vi "ini_sesion.vi"(8 "error in (no error)":errorcluster, 11 "pulse_gen_and_detect_p2p in":refnum<class "pulse_gen_and_detect_p2p.lvclass">) -> (0 "error out":errorcluster, 3 "pulse_gen_and_detect_p2p out":refnum<class "pulse_gen_and_detect_p2p.lvclass">)   [LabVIEW 2021, in "pulse_gen_and_detect_p2p.lvclass"]
uses:
  pulse_gen_and_detect_p2p.lvclass
  pulse_gen_and_detect_p2p.lvclass/pulse_gen_and_detect_p2p.ctl
  <instrlib>/niRFSG/niRFSG.llb/niRFSG Ref Clock Sources.ctl
  <instrlib>/niRFSA/niRFSA.llb/niRFSA Acquisition Types.ctl
  <vilib>/FPGAPlugInAG/PXIe-5785 (KU060)/niLvFpga_Open_PXIe-5785 (KU060).vi
  <vilib>/rvi/interface/common/dynamic/niFpgaDynamicAddResources.vi
  <vilib>/FPGAPlugInAG/Dynamic/niLvFpga_P2PGetEndpoint_Dynamic.vi
  <vilib>/Utility/error.llb/Error Cluster From Error Code.vi
  <vilib>/rvi/interface/common/niFpgaWaitOnOcc.vi
  <vilib>/rvi/errors/niLvFpgaAdjustHostInterfaceError.vi
  <vilib>/rvi/interface/nirviOpenFPGA/nirviOpenFPGA.xnode
  FPGA Bitfiles/5785_p2p_IQ_gen_1_6GHz_max_and_pulse_detector.lvbitx
  <vilib>/rvi/interface/nirviMethod/nirviMethod.xnode
  <vilib>/rvi/interface/nirviReadWriteControl/nirviReadWriteControl.xnode
  <vilib>/rvi/errors/niLvFpgaMergeErrorWithErrorCode.vi
  <vilib>/rvi/interface/Simulation/niFpgaSimulationCallBeginRW.vi
  <vilib>/FPGAPlugInAG/Dynamic/niLvFpga_StopFifo_Dynamic.vi
  <vilib>/FPGAPlugInAG/Dynamic/niLvFpga_ConfigureFifo_Dynamic.vi
  NiFpgaLv.dll
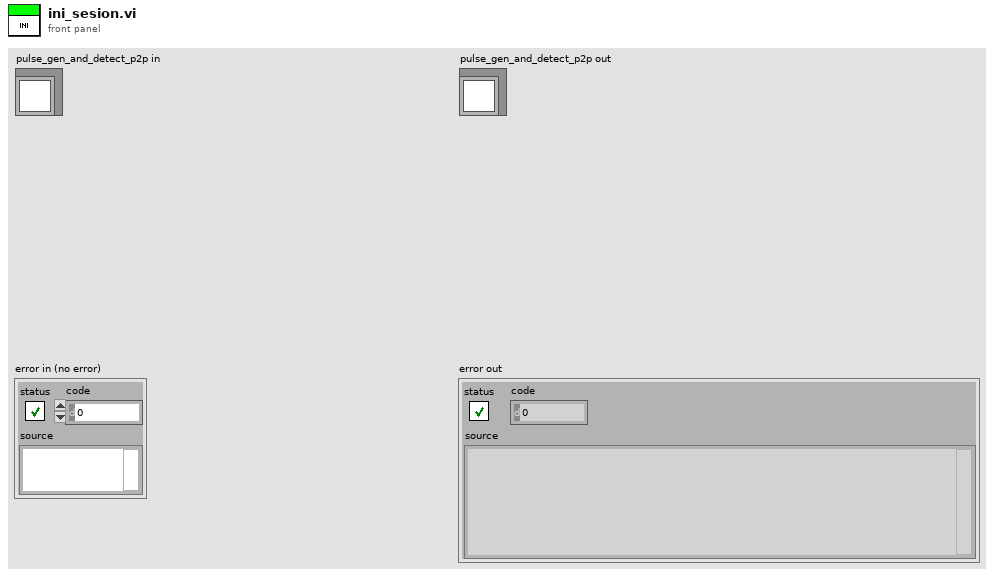
[diagram p1: front panel]
types:
  T1 = typedef "nirio_resource_hc.ctl" = tag
  T2 = cluster{"min PW (fft cycels)":u16, "max PW (fft cycels)":u16, "max gap (fft cycels)":u8, "detection bar (liniar amp)":fxp<+,64,63>, "peak detect":bool}
  T3 = enum16{"open", "open or create", "create or replace", "create", "open (read-only)"}
  T4 = typedef "niRFSG Ref Clock Sources.ctl" = string
  T5 = typedef "niRFSA Acquisition Types.ctl" = i32
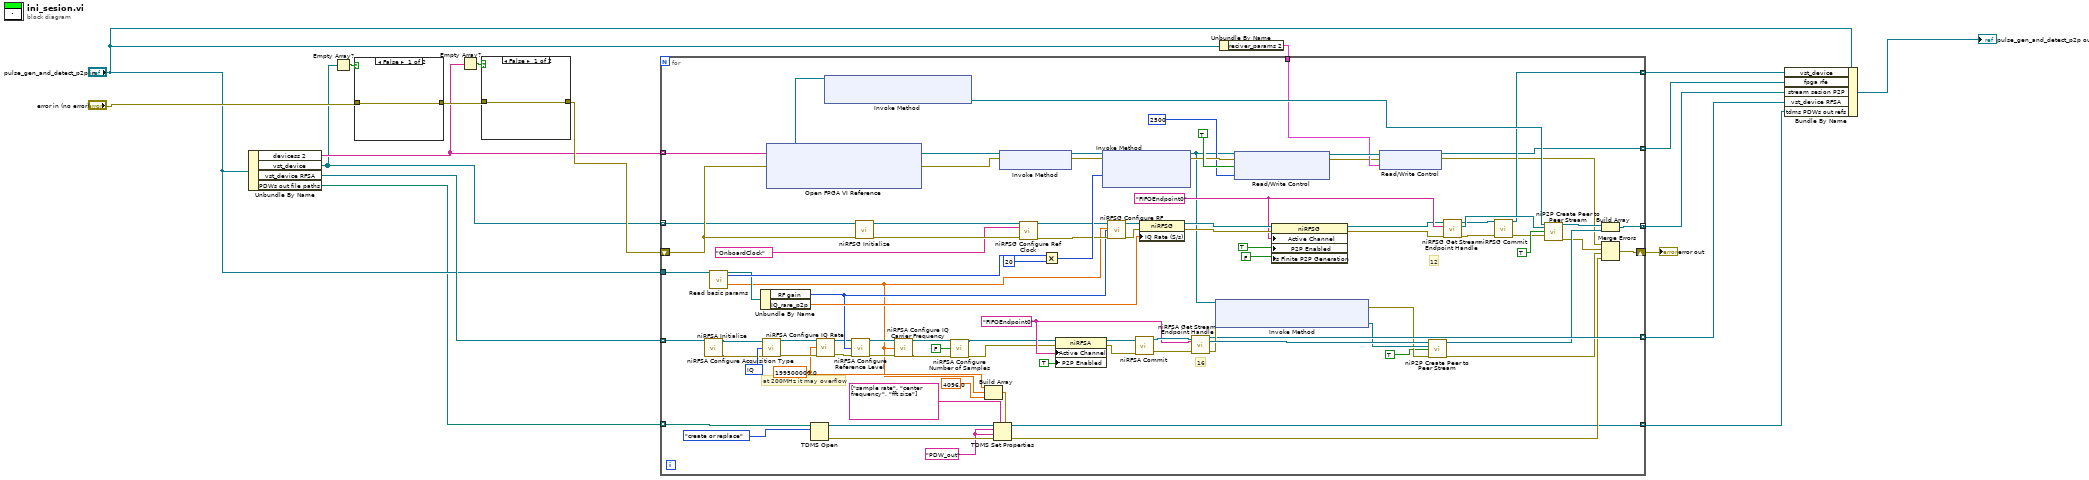
[diagram p0: block diagram]
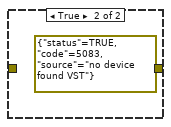
[diagram p2: hidden frame]
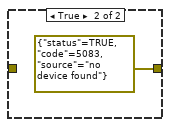
[diagram p3: hidden frame]
diagram:
  n1 = Unbundle By Name("pulse_gen_and_detect_p2p in") -> ("devicess 2"=w12:T1[], "vst_device"=w11:refnum<k15>[], "vst_device RFSA"=w7:refnum<k15>[], "PDWs out file paths"=w3:path[])
  n2 = Empty Array?(array=w11) -> (empty?=w17:bool)
  n3 = case shown="False" w17 {
    tunnel: [w19 errorcluster {"status"=TRUE, "code"=5083, "source"="no device found VST"} ("error in (no error)")] -> w16
    tunnel: "error in (no error)" -> [w19 _]
    frame False {
    }
    frame True {
    }
  }
  n4 = Empty Array?(array=w12) -> (empty?=w18:bool)
  n5 = case shown="False" w18 {
    tunnel: [w21 errorcluster {"status"=TRUE, "code"=5083, "source"="no device found"} ("error in (no error)")] -> w13
    tunnel: w16 -> [w21 _]
    frame False {
    }
    frame True {
    }
  }
  n6 = Unbundle By Name("pulse_gen_and_detect_p2p in") -> ("reciver_params 2"=w4:T2)
  n7 = for {
    tunnel: w12 -> [w78] mode=indexing
    tunnel: w11 -> [w29] mode=indexing
    tunnel: "pulse_gen_and_detect_p2p in" -> [w77]
    shift-right: [w32] -> w15
    shift-left: w13 -> [w79]
    tunnel: [w76] -> w10 mode=indexing
    tunnel: [w54] -> w9 mode=indexing
    tunnel: [w56] -> w8 mode=concatenating
    tunnel: w7 -> [w75] mode=indexing
    tunnel: [w61] -> w6 mode=indexing
    tunnel: w4 -> [w53]
    tunnel: w3 -> [w52] mode=indexing
    tunnel: [w31] -> w2 mode=indexing
    w38 = "PDW_out" ("group name")
    w42 = 199500000.0 ("IQ rate (S/s)")
    w30 = "FIFOEndpoint0" ("Active Channel")
    w74 = T5 100 items=["IQ"=100, "Spectrum"=101] ("acquisition type")
    w86 = "FIFOEndpoint0" ("format string")
    # "at 200MHz it may overflow"
    # "16"
    # "12"
    n8 = call <instrlib>:"niRFSA Initialize.vi"("resource name"=w75) -> ("instrument handle out"=w73:refnum<k15>, "error out"=w72:errorcluster)  [unwired: 13 in]
    n9 = call-dynamic "Read basic params.vi"("device_type in"=w77) -> ("device_type out"=w81:refnum<class "pulse_gen_and_detect_p2p.lvclass">, "buffer size"=w82:u32, "center frequency (Hz)"=w41:dbl)  [unwired: 13 in, 3 out]
    n10 = Unbundle By Name(w81) -> ("RF gain"=w71:i32, "IQ_rare_p2p"=w90:dbl)
    n11 = call <instrlib>:"niRFSA Configure Acquisition Type.vi"("instrument handle"=w73, "acquisition type"=w74, "error in"=w72) -> ("instrument handle out"=w48:refnum<k15>, "error out"=w45:errorcluster)  [unwired: 11 in]
    n12 = xnode "Open FPGA VI Reference"("error in"=w79, "resource name"=w78) -> ("FPGA VI Reference Out"=w100:refnum<k20>, "error out"=w109:errorcluster)
    n13 = TDMS Open(10:T3."create or replace" ("operation (0:open)"), 11:w52) -> (0:w49:errorcluster, 3:w50:refnum<k34>)  [unwired: 5 in]
    n14 = call <instrlib>:"niRFSA Configure IQ Rate.vi"("instrument handle"=w48, "IQ rate (S/s)"=w42, "error in"=w45) -> ("instrument handle out"=w47:refnum<k15>, "error out"=w46:errorcluster)  [unwired: 11 in]
    n15 = xnode "Invoke Method"("FPGA VI Reference In"=w100) -> ("Writer"=w80:refnum<k20>)  [unwired: 1 in, 2 out]
    n16 = call <instrlib>:"niRFSA Configure Reference Level.vi"("instrument handle"=w47, "reference level (dBm)"=w71, "error in"=w46) -> ("instrument handle out"=w70:refnum<k15>, "error out"=w69:errorcluster)  [unwired: 11 in]
    n17 = call <instrlib>:"niRFSG Initialize.vi"("resource name"=w29, "error in"=w79) -> ("instrument handle"=w104:refnum<k15>, "error out"=w103:errorcluster)  [unwired: 12 in]
    n18 = call <instrlib>:"niRFSA Configure IQ Carrier Frequency.vi"("instrument handle"=w70, "carrier frequency"=w41, "error in"=w69) -> ("instrument handle out"=w26:refnum<k15>, "error out"=w25:errorcluster)  [unwired: 11 in]
    n19 = call <instrlib>:"niRFSA Configure Number of Samples.vi"("instrument handle"=w26, "number of samples is finite"=FALSE, "error in"=w25) -> ("instrument handle out"=w24:refnum<k15>, "error out"=w23:errorcluster)  [unwired: 11 in]
    n20 = Build Array(w42, w41, 4096.0 ("element")) -> (w39:dbl[])
    n21 = TDMS Set Properties(5:w39, 7:string[] ["sample rate", "center frequency", "fft size"] ("property names"), 8:w49, 9:w38, 10:w38, 11:w50) -> (0:w36:errorcluster, 3:w31:refnum<k34>)  [unwired: 2 out]
    n22 = xnode "Invoke Method"("FPGA VI Reference In"=w100, "error in"=w109) -> ("FPGA VI Reference Out"=w107:refnum<k20>, "error out"=w108:errorcluster)
    n23 = call <instrlib>:"niRFSG Configure Ref Clock.vi"("instrument handle"=w104, "ref clock source"=T4 "OnboardClock", "error in"=w103) -> ("instrument handle out"=w96:refnum<k15>, "error out"=w95:errorcluster)  [unwired: 11 in]
    n24 = Multiply(x=w82, y=u32 20) -> (x*y=w111:u32)
    n25 = property class="niRFSA"(reference=w24, error in=w23, "Active Channel"=w30, "P2P Enabled"=TRUE ("Peer-to-Peer:Enabled")) -> (reference out=w68:refnum<k15>, error out=w67:errorcluster)
    n26 = xnode "Invoke Method"("FPGA VI Reference In"=w107, "error in"=w108, "Requested Depth"=w111) -> ("FPGA VI Reference Out"=w63:refnum<k20>, "error out"=w105:errorcluster)  [unwired: 1 out]
    n27 = call <instrlib>:"niRFSG Configure RF.vi"("instrument handle"=w96, "frequency (Hz)"=w41, "power level (dBm)"=w71, "error in"=w95) -> ("instrument handle out"=w94:refnum<k15>, "error out"=w93:errorcluster)  [unwired: 10 in]
    n28 = call <instrlib>:"niRFSA Commit.vi"("instrument handle"=w68, "error in"=w67) -> ("instrument handle out"=w66:refnum<k15>, "error out"=w65:errorcluster)  [unwired: 12 in]
    n29 = property class="niRFSG"(reference=w94, error in=w93, "IQ Rate (S/s)"=w90) -> (reference out=w92:refnum<k15>, error out=w91:errorcluster)
    n30 = call <instrlib>:"niRFSA Get Stream Endpoint Handle.vi"("instrument handle"=w66, "stream endpoint"=w30, "error in"=w65) -> ("instrument handle out"=w61:refnum<k15>, "writer handle"=w64:refnum<k20>, "error out"=w62:errorcluster)  [unwired: 10 in]
    n31 = xnode "Invoke Method"("FPGA VI Reference In"=w63, "error in"=w62) -> ("error out"=w59:errorcluster, "Reader"=w60:refnum<k20>)  [unwired: 1 out]
    n32 = xnode "Read/Write Control"("FPGA VI Reference In"=w63, "error in"=w105, "reset system clock"=TRUE, "P2P empty room for runing"=u32 2500) -> ("FPGA VI Reference Out"=w55:refnum<k20>, "error out"=w37:errorcluster)
    n33 = property class="niRFSG"(reference=w92, error in=w91, "Active Channel"=w86, "P2P Enabled"=TRUE ("Peer-to-Peer:Enabled"), "Is Finite P2P Generation"=FALSE ("Peer-to-Peer:Is Finite Generation")) -> (reference out=w85:refnum<k15>, error out=w84:errorcluster)
    n34 = xnode "Read/Write Control"("FPGA VI Reference In"=w55, "error in"=w37, "reciver_params 2"=w53) -> ("FPGA VI Reference Out"=w54:refnum<k20>, "error out"=w33:errorcluster)
    n35 = call <vilib>:"niP2P Create Peer to Peer Stream.vi"("writer"=w64, "reader"=w60, "enable stream (T)"=TRUE, "error in (no error)"=w59) -> ("stream session"=w57:refnum<k20>, "error out"=w35:errorcluster)  [unwired: 10 in]
    n36 = call <instrlib>:"niRFSG Get Stream Endpoint Handle.vi"("instrument handle"=w85, "stream endpoint"=w86, "error in"=w84) -> ("instrument handle out"=w89:refnum<k15>, "reader handle"=w101:refnum<k20>, "error out"=w88:errorcluster)  [unwired: 10 in]
    n37 = call <instrlib>:"niRFSG Commit.vi"("instrument handle"=w89, "error in"=w88) -> ("instrument handle out"=w76:refnum<k15>, "error out"=w87:errorcluster)  [unwired: 12 in]
    n38 = call <vilib>:"niP2P Create Peer to Peer Stream.vi"("writer"=w80, "reader"=w101, "enable stream (T)"=TRUE, "error in (no error)"=w87) -> ("stream session"=w58:refnum<k20>, "error out"=w34:errorcluster)  [unwired: 10 in]
    n39 = Build Array(w58, w57) -> (w56:refnum<k20>[])
    n40 = Merge Errors(w33, w34, w35, w36) -> (w32:errorcluster)
  }
  "error out" <- w15
  n41 = Bundle By Name(cluster="pulse_gen_and_detect_p2p in", "vst_device"=w10, "fpga rfe"=w9, "stream sesion P2P"=w8, "vst_device RFSA"=w6, "tdms PDWs out refs"=w2) -> (→"pulse_gen_and_detect_p2p out":refnum<class "pulse_gen_and_detect_p2p.lvclass">)
